vi "Parse Measurement.vi"(0 "Labeling (off)":bool, 1 "Sample Field (on)":bool=TRUE, 2 "Frequency Field (on)":bool=TRUE, 3 "Capacitance Field (9)":i32=9 min=0 max=9, 4 "Loss Field (9)":i32=9 min=0 max=9, 5 "Voltage Field (on)":bool=TRUE, 6 "Measurement Line":string, 7 "Error Messages (off)":bool) -> (11 "Error Message":string, 12 "Error Code":i32, 13 "Voltage":dbl, 14 "Sample":i32, 15 "Frequency":dbl, 16 "Capacitance":dbl format="%#_10f", 17 "Loss":dbl format="%#_10f", 18 "Units":i32(ring) items=["", "nanosiemens", "dissipation factor", "kilohms", "gigohms", "loss vector (jpF)"], 19 "Loss Greater Than":bool)   [LabVIEW 2016, in "Andeen-Hagerling 2700.lvlib"]
doc: "This VI parses a text line of measurement results from the bridge. Measurement results are dependent on the labelling parameter of Format and the Field parameters. Boolean inputs are provided to represent these parameters. These only need to be set if the the Format or Field are not set as in the Default Instrument Setup VI."
uses:
  Andeen-Hagerling 2700.lvlib
panel:
  # "Measurement Results"
  # "Format Parameter"
  # "Field Parameters"
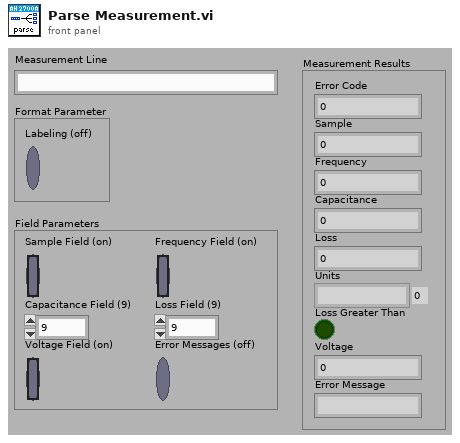
[diagram p1: front panel]
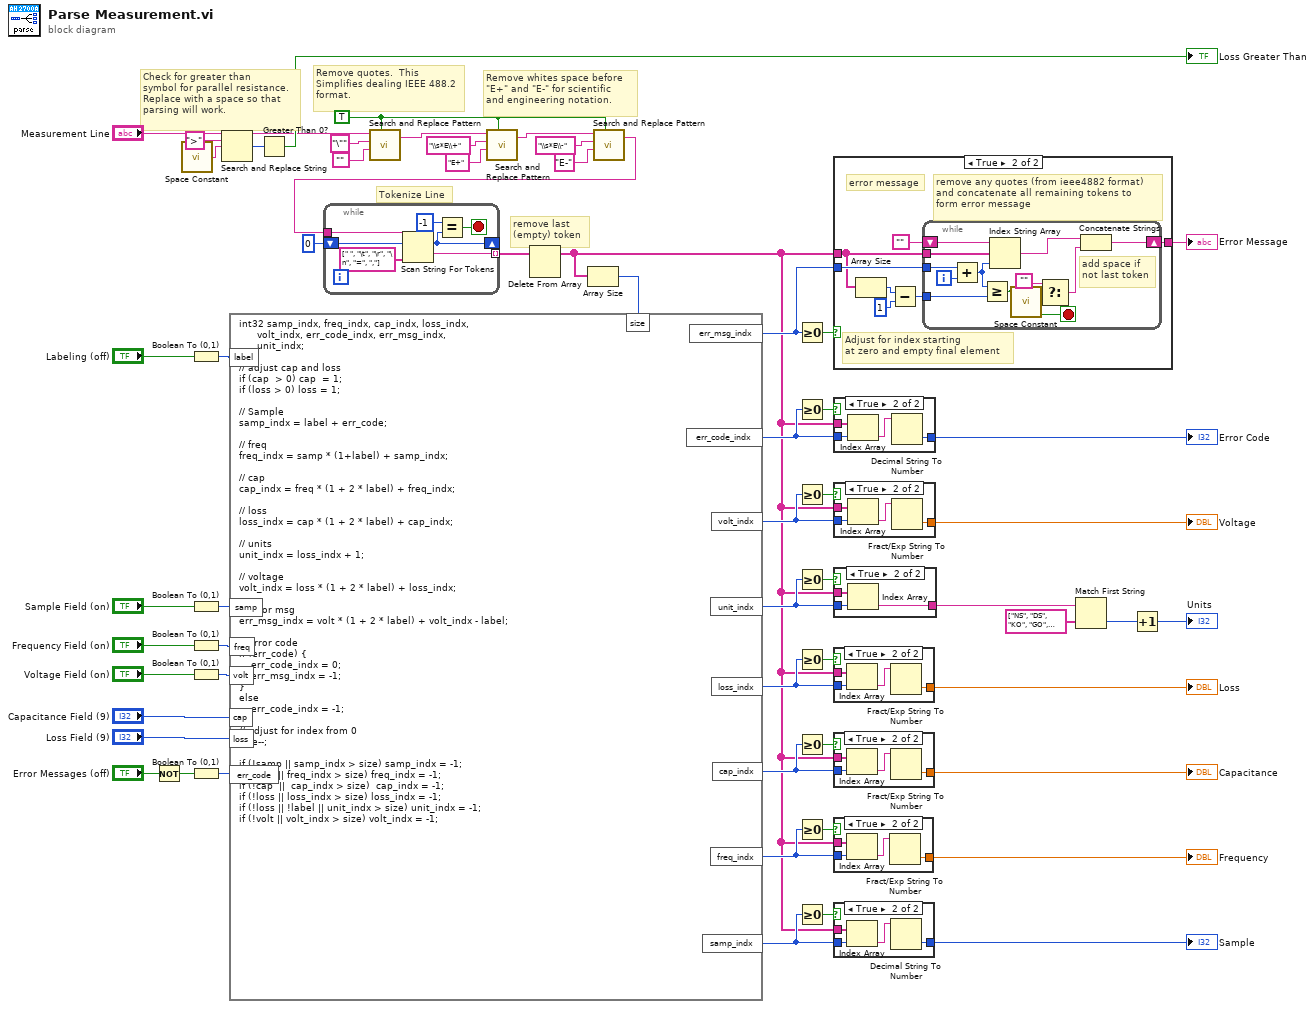
[diagram p0: block diagram]
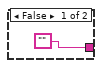
[diagram p2: hidden frame]
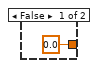
[diagram p3: hidden frame]
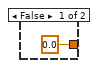
[diagram p4: hidden frame]
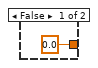
[diagram p5: hidden frame]
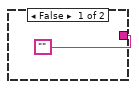
[diagram p6: hidden frame]
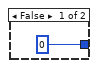
[diagram p7: hidden frame]
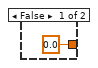
[diagram p8: hidden frame]
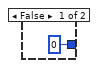
[diagram p9: hidden frame]
diagram:
  w5 = TRUE ("replace all? (F)")
  # "remove last\n(empty) token"
  # "Remove quotes.  This\nSimplifies dealing IEEE 488.2\nformat."
  # "Remove whites space before\n\"E+\" and \"E-\" for scientific\nand engineering notation."
  # "Tokenize Line"
  # "Check for greater than\nsymbol for parallel resistance.\nReplace with a space so that\nparsing will work."
  n1 = Not(x="Error Messages (off)") -> (.not. x?=w29:bool)
  n2 = call <vilib>:"Space Constant.vi"() -> ("String"=w53:string)
  n3 = Boolean To (0,1)(Boolean="Labeling (off)") -> (0, 1=w31:i16)
  n4 = Boolean To (0,1)(Boolean="Sample Field (on)") -> (0, 1=w27:i16)
  n5 = Boolean To (0,1)(Boolean="Frequency Field (on)") -> (0, 1=w25:i16)
  n6 = Boolean To (0,1)(Boolean="Voltage Field (on)") -> (0, 1=w24:i16)
  n7 = Boolean To (0,1)(Boolean=w29) -> (0, 1=w30:i16)
  n8 = Search and Replace String(input string="Measurement Line", search string=">", replace string=w53) -> (result string=w2:string, number of replacements=w54:i32)  [unwired: 5 in, 2 out]
  n9 = Greater Than 0?(x=w54) -> (x > 0?=→"Loss Greater Than":bool)
  n10 = call <vilib>:"Search and Replace Pattern.vi"("string"=w2, "regular expression (\"\")"="\"" ("regular expression (\"\")"), "replace string (\"\")"="", "replace all? (F)"=w5) -> ("result string"=w8:string)  [unwired: 1 in, 1 out]
  n11 = call <vilib>:"Search and Replace Pattern.vi"("string"=w8, "regular expression (\"\")"="\\s*E\\+" ("regular expression (\"\")"), "replace string (\"\")"="E+" ("replace string (\"\")"), "replace all? (F)"=w5) -> ("result string"=w9:string)  [unwired: 1 in, 1 out]
  n12 = call <vilib>:"Search and Replace Pattern.vi"("string"=w9, "regular expression (\"\")"="\\s*E\\-" ("regular expression (\"\")"), "replace string (\"\")"="E-" ("replace string (\"\")"), "replace all? (F)"=w5) -> ("result string"=w1:string)  [unwired: 1 in, 1 out]
  n13 = while {
    tunnel: [w66] -> w4 mode=indexing
    tunnel: w1 -> [w65]
    shift-right: [w63] -> _
    shift-left: 0 ("token index") -> [w64]
    stop <- w67 stop-if-true
    n14 = Scan String For Tokens(6:string[] [" ", "\t", "\r", "\n", "=", ","] ("delimiters (\\s,\\t,\\r,\\n)"), 8:w64, 9:w65) -> (1:w66:string, 2:w63:i32)  [unwired: 3 in, 2 out]
    n15 = Equal?(x=-1 ("y"), y=w63) -> (x = y?=w67:bool)
  }
  n16 = Delete From Array(array=w4) -> (array with subset deleted=w3:string[])  [unwired: 2 in, 1 out]
  n17 = Array Size(array=w3) -> (size(s)=w34:i32)
  n18 = formula code="int32 samp_indx, freq_indx, cap_indx, loss_indx, \n      volt_indx, err_code_indx, err_msg_indx,\n      unit_indx;\n\n// adjust cap and loss\nif (cap  > 0) cap  = 1;\nif (loss > 0) loss = 1;\n\n// Sample\nsamp_indx = label + err_code;\n\n// freq\nfreq_indx = samp * (1+label) + samp_indx;\n\n// cap\ncap_indx = freq * (1 + 2 * label) + freq_indx;\n\n// loss\nloss_indx = cap * (1 + 2 * label) + cap_indx;\n\n// units\nunit_indx = loss_indx + 1;\n\n// voltage\nvolt_indx = loss * (1 + 2 * label) + loss_indx;\n\n// Error msg\nerr_msg_indx = volt * (1 + 2 * label) + volt_indx - label;\n\n// Error code\nif (err_code) {\n    err_code_indx = 0;\n    err_msg_indx = -1;\n}\nelse\n    err_code_indx = -1;\n\n// adjust for index from 0\nsize--;\n\nif (!samp || samp_indx > size) samp_indx = -1;\nif (!freq || freq_indx > size) freq_indx = -1;\nif (!cap  ||  cap_indx > size)  cap_indx = -1;\nif (!loss || loss_indx > size) loss_indx = -1;\nif (!loss || !label || unit_indx > size) unit_indx = -1;\nif (!volt || volt_indx > size) volt_indx = -1;"("samp"=w27, "label"=w31, "err_code"=w30, "freq"=w25, "cap"="Capacitance Field (9)", "loss"="Loss Field (9)", "volt"=w24, "size"=w34) -> ("cap_indx"=w51:i32, "freq_indx"=w52:i32, "loss_indx"=w50:i32, "samp_indx"=w58:i32, "volt_indx"=w49:i32, "err_code_indx"=w57:i32, "err_msg_indx"=w56:i32, "unit_indx"=w48:i32)
  n19 = Greater Or Equal To 0?(x=w56) -> (x >= 0?=w40:bool)
  n20 = Greater Or Equal To 0?(x=w57) -> (x >= 0?=w41:bool)
  n21 = Greater Or Equal To 0?(x=w49) -> (x >= 0?=w39:bool)
  n22 = Greater Or Equal To 0?(x=w48) -> (x >= 0?=w42:bool)
  n23 = Greater Or Equal To 0?(x=w50) -> (x >= 0?=w43:bool)
  n24 = Greater Or Equal To 0?(x=w51) -> (x >= 0?=w38:bool)
  n25 = Greater Or Equal To 0?(x=w52) -> (x >= 0?=w37:bool)
  n26 = Greater Or Equal To 0?(x=w58) -> (x >= 0?=w44:bool)
  n27 = case shown="True" w40 {
    tunnel: w3 -> [_ w74]
    tunnel: w56 -> [_ w75]
    tunnel: ["" w73] -> w60
    frame False {
    }
    frame True {
      # "Adjust for index starting\nat zero and empty final element"
      # "error message"
      # "remove any quotes (from ieee4882 format)\nand concatenate all remaining tokens to \nform error message"
      n28 = Array Size(array=w74) -> (size(s)=w71:i32)
      n29 = Subtract(x=w71, y=1) -> (x-y=w72:i32)
      n30 = while {
        tunnel: w75 -> [w86]
        tunnel: w74 -> [w87]
        tunnel: w72 -> [w83]
        shift-right: [w82] -> w73
        shift-left: "" -> [w77]
        i -> [w85]
        stop <- w78 stop-if-true
        # "add space if\nnot last token"
        n31 = Add(x=w86, y=w85) -> (x+y=w84:i32)
        n32 = Greater Or Equal?(x=w84, y=w83) -> (x >= y?=w78:bool)
        n33 = Index String Array(1:w84, 2:w87, 3:w77) -> (0:w76:string)
        n34 = call <vilib>:"Space Constant.vi"() -> ("String"=w79:string)
        n35 = Select(t="", s=w78, f=w79) -> (s? t:f=w80:string)
        n36 = Concatenate Strings(w76, w80) -> (w82:string)
      }
    }
  }
  "Error Message" <- w60
  n37 = case shown="True" w41 {
    tunnel: w3 -> [_ w92]
    tunnel: w57 -> [_ w90]
    tunnel: [0 w89] -> w59
    frame False {
    }
    frame True {
      n38 = Index Array(array=w92, index=w90) -> (element=w91:string)
      n39 = Decimal String To Number(string=w91) -> (number=w89:i32)  [unwired: 2 in, 1 out]
    }
  }
  "Error Code" <- w59
  n40 = case shown="True" w39 {
    tunnel: w3 -> [_ w96]
    tunnel: w49 -> [_ w95]
    tunnel: [0.0 w97] -> w21
    frame False {
    }
    frame True {
      n41 = Index Array(array=w96, index=w95) -> (element=w94:string)
      n42 = Fract/Exp String To Number(string=w94) -> (number=w97:dbl)  [unwired: 3 in, 1 out]
    }
  }
  "Voltage" <- w21
  n43 = case shown="True" w42 {
    tunnel: w3 -> [_ w101]
    tunnel: w48 -> [_ w100]
    tunnel: ["" w99] -> w20
    frame False {
    }
    frame True {
      n44 = Index Array(array=w101, index=w100) -> (element=w99:string)
    }
  }
  n45 = case shown="True" w43 {
    tunnel: w3 -> [_ w105]
    tunnel: w50 -> [_ w104]
    tunnel: [0.0 w106] -> w45
    frame False {
    }
    frame True {
      n46 = Index Array(array=w105, index=w104) -> (element=w103:string)
      n47 = Fract/Exp String To Number(string=w103) -> (number=w106:dbl)  [unwired: 3 in, 1 out]
    }
  }
  "Loss" <- w45
  n48 = case shown="True" w38 {
    tunnel: w3 -> [_ w110]
    tunnel: w51 -> [_ w109]
    tunnel: [0.0 w111] -> w46
    frame False {
    }
    frame True {
      n49 = Index Array(array=w110, index=w109) -> (element=w108:string)
      n50 = Fract/Exp String To Number(string=w108) -> (number=w111:dbl)  [unwired: 3 in, 1 out]
    }
  }
  "Capacitance" <- w46
  n51 = case shown="True" w37 {
    tunnel: w3 -> [_ w115]
    tunnel: w52 -> [_ w114]
    tunnel: [0.0 w116] -> w36
    frame False {
    }
    frame True {
      n52 = Index Array(array=w115, index=w114) -> (element=w113:string)
      n53 = Fract/Exp String To Number(string=w113) -> (number=w116:dbl)  [unwired: 3 in, 1 out]
    }
  }
  "Frequency" <- w36
  n54 = case shown="True" w44 {
    tunnel: w3 -> [_ w121]
    tunnel: w58 -> [_ w120]
    tunnel: [0 w118] -> w47
    frame False {
    }
    frame True {
      n55 = Index Array(array=w121, index=w120) -> (element=w119:string)
      n56 = Decimal String To Number(string=w119) -> (number=w118:i32)  [unwired: 2 in, 1 out]
    }
  }
  "Sample" <- w47
  n57 = Match First String(2:string[] ["NS", "DS", "KO", "GO", "JP"] ("string array"), 3:w20) -> (0:w18:i32)  [unwired: 1 out]
  n58 = Increment(x=w18) -> (x+1=→"Units":i32)
